vi "Actor Core.vi"(8 "error in":errorcluster, 11 "Main in":refnum<class "Main.lvclass">) -> (0 "error out":errorcluster, 3 "Actor out":refnum<class "Actor.lvclass">)   [LabVIEW 2015, in "Main.lvlib" / "Main.lvclass"]
doc: "(<B>Filename</B>: Actor Framework.lvlib:Actor.lvclass:Actor Core.vi)\n\nReceives messages to the actor, reacts to them, and initiates any error handling that may shut the actor down.\n\nDescendant classes may override this VI to append parallel tasks for the actor to complete while it handles messages. Overrides use the Call Parent Method node."
uses:
  Main.lvclass
  <vilib>/ActorFramework/Actor/Actor.lvclass
  <vilib>/ActorFramework/Actor/Actor.lvclass/Actor.ctl
  <vilib>/ActorFramework/Message Enqueuer/Message Enqueuer.lvclass/Message Enqueuer.ctl
  Main.lvclass/Main.ctl
  Main Messages/Method Msg/Method Msg.lvclass/Method Msg.ctl
  <vilib>/ActorFramework/Message Enqueuer/Init from Existing Queue.vi
  <vilib>/ActorFramework/Message Enqueuer/Enqueue.vi
  <vilib>/ActorFramework/Message Priority Queue/Priority Enqueue.vi
  <vilib>/ActorFramework/Message Enqueuer/Message Enqueuer.lvclass
  <vilib>/ActorFramework/Stop Msg/Stop Msg.lvclass
  Main Messages/Method Msg/Method Msg.lvclass
panel:
  in  "Trigger":bool
  in  "Numeric":dbl=1001.0
  in  "String":string="Message"
  in  "stop":bool
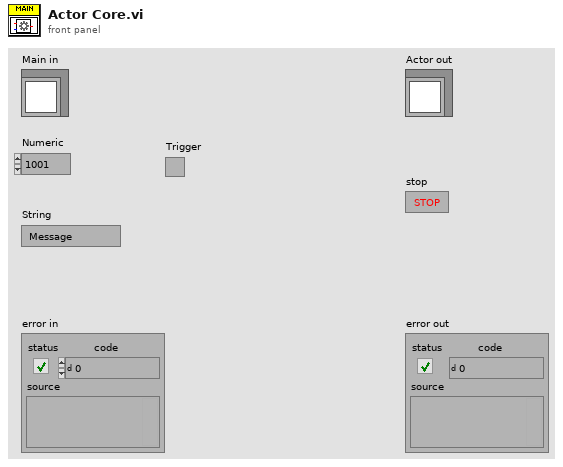
[diagram p1: front panel]
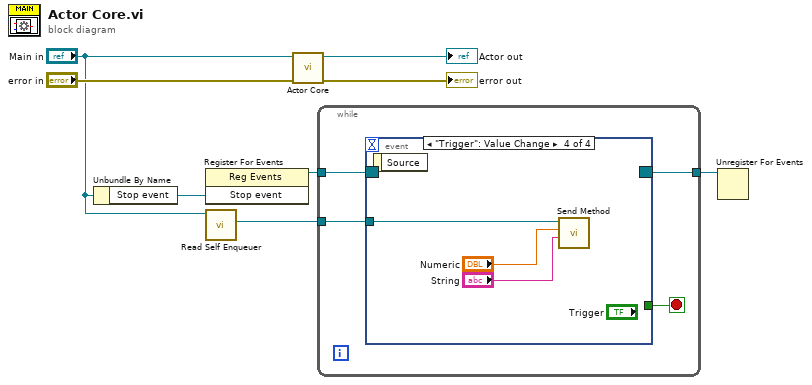
[diagram p0: block diagram]
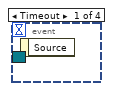
[diagram p2: hidden frame]
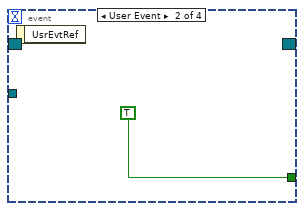
[diagram p3: hidden frame]
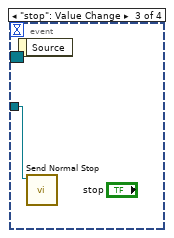
[diagram p4: hidden frame]
diagram:
  n1 = Unbundle By Name("Main in") -> ("Stop event"=w3:refnum<user-event>)
  n2 = register-events(w3) -> (reference out=w4:refnum<event-registration>)  [unwired: 2 in, 1 out]
  n3 = call <vilib>:"Read Self Enqueuer.vi"("Actor"="Main in") -> ("Self Enqueuer"=w2:refnum<class "Message Enqueuer.lvclass">)  [unwired: 10 in]
  n4 = call-parent "Actor Core.vi"("error in"="error in", "Actor in"="Main in") -> ("error out"=→"error out":errorcluster, "Actor out"=→"Actor out":refnum<class "Actor.lvclass">)  [unwired: 8 in]
  n5 = while {
    tunnel: w2 -> [w12]
    tunnel: w4 -> [w11]
    tunnel: [w9] -> w5
    stop <- w10 stop-if-true
    n6 = event shown="[3] \"Trigger\": Value Change" {
      selector: w11 -> [_ _ _ _]
      dyn-events: [_ _ _ _] -> w9
      timeout: _ -> [_ _ _ _]
      tunnel: w12 -> [_ _ w14 w15]
      tunnel: [_ TRUE _ _] -> w10
      event Timeout {
        n7 = event-data() -> ()  [unwired: 1 in, 1 out]
      }
      event User Event {
        n8 = event-data() -> ()  [unwired: 1 in, 1 out]
      }
      event "stop": Value Change {
        n9 = event-data() -> ()  [unwired: 1 in, 1 out]
        n10 = call <vilib>:"Send Normal Stop.vi"("Message Enqueuer"=w14) -> ()  [unwired: 10 in, 1 out]
      }
      event "Trigger": Value Change {
        n11 = event-data() -> ()  [unwired: 1 in, 1 out]
        n12 = call "Send Method.vi"("String"="String", "Numeric"="Numeric", "Message Enqueuer"=w15) -> ()  [unwired: 7 in, 2 out]
      }
    }
  }
  n13 = Unregister For Events(event registration refnum=w5) -> ()  [unwired: 1 in, 1 out]
